vi "Randomize Array (LabVIEW 2016).vi"() -> ()   [LabVIEW 2016]
panel:
  out "Randomized Array":string[](array[string])
  in  "Input Array":string[](array[string])
  # "Overview: This VI will randomize the order of Input Array elements\nRequirements: LabVIEW 2012 (or compatible)\nInstructions:\n1. Manually Initialize the Input Array\n2. Run the VI"
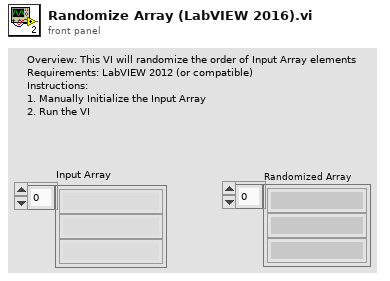
[diagram p1: front panel]
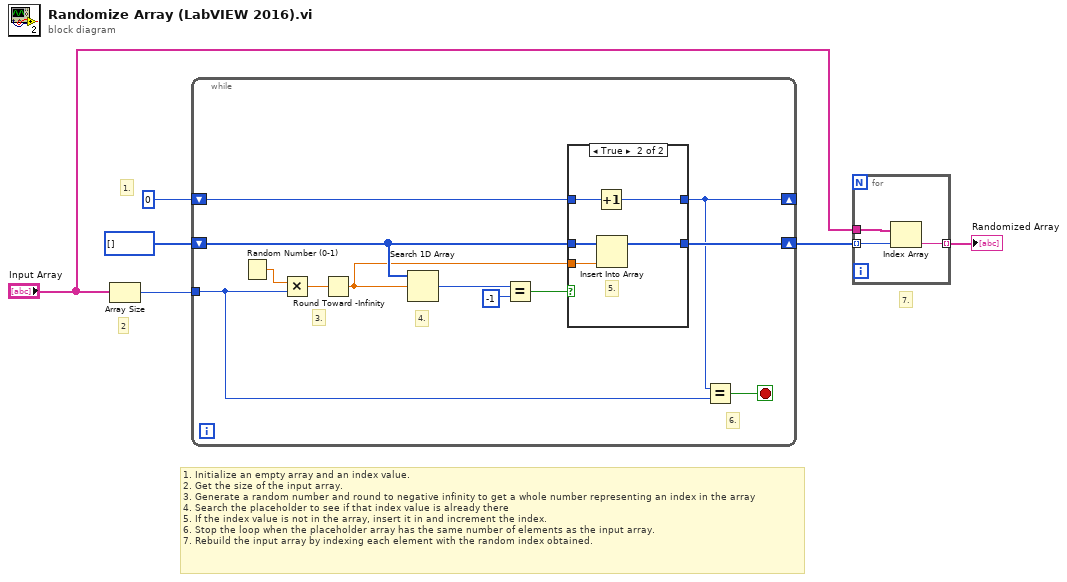
[diagram p0: block diagram]
diagram:
  # "1. Initialize an empty array and an index value.\n2. Get the size of the input array.\n3. Generate a random number and round to negative infinity to get a whole number representing an index in the array\n4. Search the placeholder to see if that index value is already there\n5. If the index value is not in the array, insert it in and increment the index.\n6. Stop the loop when the placeholder array has the same number of elements as the input array.\n7. Rebuild the input array by indexing each element with the random index obtained."
  # "7."
  # "2"
  # "1."
  n1 = Array Size(array="Input Array") -> (size(s)=w6:i32)
  n2 = while {
    tunnel: w6 -> [w10]
    shift-right: [w9] -> _
    shift-left: 0 -> [w15]
    shift-right: [w14] -> w3
    shift-left: i32[] [] -> [w11]
    stop <- w16 stop-if-true
    # "6."
    # "4."
    # "3."
    n3 = Random Number (0-1)() -> (number: 0 to 1=w8:dbl)
    n4 = Multiply(x=w8, y=w10) -> (x*y=w12:dbl)
    n5 = Round Toward -Infinity(1:w12) -> (0:w7:dbl)
    n6 = Search 1D Array(1D array=w11, element=w7) -> (index of element=w18:i32)  [unwired: 1 in]
    n7 = Equal?(x=w18, y=-1) -> (x = y?=w17:bool)
    n8 = case shown="True" w17 {
      tunnel: w15 -> [w20 w25]
      tunnel: [w20 w24] -> w9
      tunnel: w11 -> [w19 w23]
      tunnel: [w19 w22] -> w14
      tunnel: w7 -> [_ w21]
      frame False {
      }
      frame True {
        # "5."
        n9 = Increment(x=w25) -> (x+1=w24:i32)
        n10 = Insert Into Array(array=w23, new element=w21) -> (w22:i32[])  [unwired: 1 in]
      }
    }
    n11 = Equal?(x=w9, y=w10) -> (x = y?=w16:bool)
  }
  n12 = for {
    tunnel: w3 -> [w28] mode=indexing
    tunnel: "Input Array" -> [w27]
    tunnel: [w26] -> w2 mode=indexing
    n13 = Index Array(array=w27, index=w28) -> (element=w26:string)
  }
  "Randomized Array" <- w2
